vi "publish.vi"(0 "HGF_DSCService":refnum<class "HGF_DSCService.lvclass">, 1 "typeDescriptor":string, 2 "data":variant, 3 "timeout in ms (-1)":i32, 5 "error in (no error)":errorcluster) -> (14 "dup HGF_DSCService":refnum<class "HGF_DSCService.lvclass">, 16 "rawData":variant, 17 "timed out?":bool, 19 "error out":errorcluster)   [LabVIEW 2012, in "HGF_DSC.lvlib" / "HGF_DSCService.lvclass"]
uses:
  HGF_DSCService.lvclass
  HGF_SV/HGF_SVService/HGF_SVService.lvclass
  HGF_DSCService.lvclass/HGF_DSCService.ctl
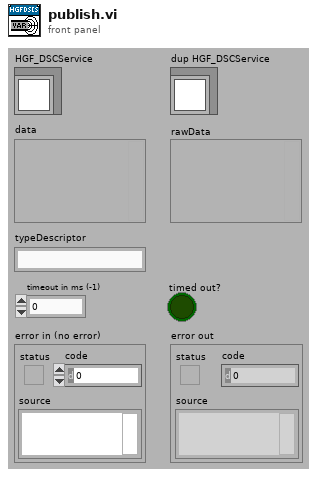
[diagram p1: front panel]
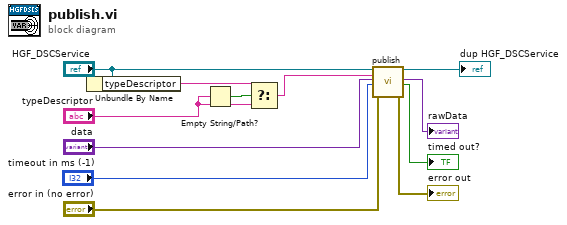
[diagram p0: block diagram]
diagram:
  n1 = Unbundle By Name("HGF_DSCService") -> ("typeDescriptor"=w4:string)
  n2 = Empty String/Path?(string/path="typeDescriptor") -> (empty?=w5:bool)
  n3 = Select(t=w4, s=w5, f="typeDescriptor") -> (s? t:f=w3:string)
  n4 = call-parent "publish.vi"("HGF_SVService"="HGF_DSCService", "typeDescriptor"=w3, "data"="data", "timeout in ms (-1)"="timeout in ms (-1)", "error in (no error)"="error in (no error)") -> ("dup HGF_SVService"=→"dup HGF_DSCService":refnum<class "HGF_DSCService.lvclass">, "rawData"=→"rawData":variant, "timed out?"=→"timed out?":bool, "error out"=→"error out":errorcluster)  [unwired: 11 out]
